vi "Keithley24xx_ConfOut2.vi"(4 "Output Type  (0: Immediate)":u16(ring) items=["Immediate", "Triggered"], 5 "Source Mode  (0: Voltage)":u16(ring) items=["Voltage", "Current"], 6 "error in (no error)":errorcluster, 7 "Compliance  Level (0.1)":dbl=0.1, 8 "Output Level (0)":dbl, 9 "VISA resource name":refnum<visa-resource-name>) -> (0 "error out":errorcluster, 3 "VISA resource name out":refnum<visa-resource-name>)   [LabVIEW 2014]
uses:
  Keithley 24XX/Keithley 24XX.lvlib
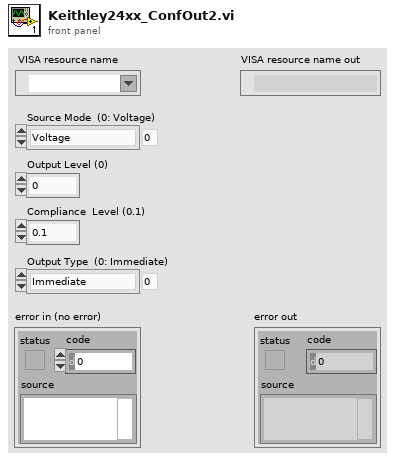
[diagram p1: front panel]
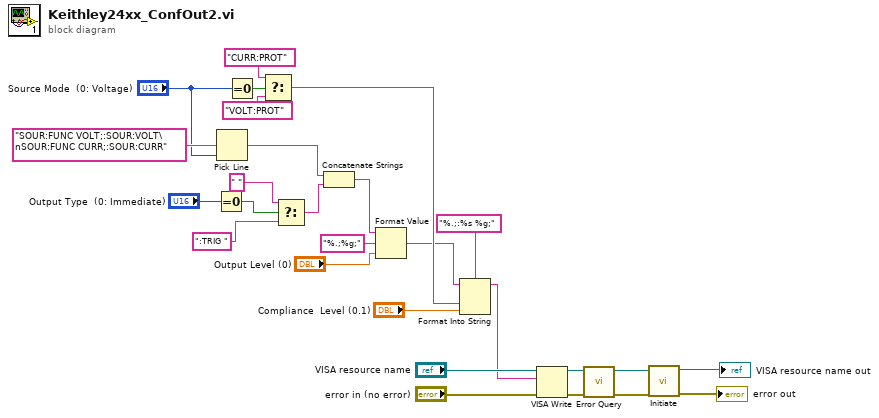
[diagram p0: block diagram]
diagram:
  n1 = Equal To 0?(x="Output Type  (0: Immediate)") -> (x = 0?=w19:bool)
  n2 = Pick Line(multi-line string="SOUR:FUNC VOLT;:SOUR:VOLT\nSOUR:FUNC CURR;:SOUR:CURR", line index="Source Mode  (0: Voltage)") -> (output string=w15:string)  [unwired: 1 in]
  n3 = Equal To 0?(x="Source Mode  (0: Voltage)") -> (x = 0?=w12:bool)
  n4 = Select(t="CURR:PROT", s=w12, f="VOLT:PROT") -> (s? t:f=w9:string)
  n5 = Select(t=" ", s=w19, f=":TRIG ") -> (s? t:f=w16:string)
  n6 = Concatenate Strings(w15, w16) -> (w14:string)
  n7 = Format Value(string ("")=w14, format string="%.;%g;", value (0)="Output Level (0)") -> (output string=w7:string)
  n8 = Format Into String(format string="%.;:%s %g;", initial string=w7, w9, "Compliance  Level (0.1)") -> (resulting string=w6:string)  [unwired: 1 in, 1 out]
  n9 = VISA Write(VISA resource name="VISA resource name", write buffer=w6, error in (no error)="error in (no error)") -> (VISA resource name out=w25:refnum<visa-resource-name>, error out=w24:errorcluster)  [unwired: 1 out]
  n10 = call "Error Query.vi"("error in (no error)"=w24, "VISA resource name"=w25) -> ("error out"=w3:errorcluster, "VISA resource name out"=w4:refnum<visa-resource-name>)  [unwired: 6 in, 2 out]
  n11 = call "Initiate.vi"("error in (no error)"=w3, "VISA resource name"=w4) -> ("error out"=→"error out":errorcluster, "VISA resource name out"=→"VISA resource name out":refnum<visa-resource-name>)  [unwired: 8 in]
